vi "Client - Child 1 -  GET.vi"(8 "error in":errorcluster) -> (0 "error out":errorcluster, 2 "value":dbl)   [LabVIEW 2023, in "Client.lvlib" / "Client.lvclass"]
uses:
  Client.lvclass
  Child_1/Usr Ev/Child_1 - Ctrl - Enum - Events.ctl
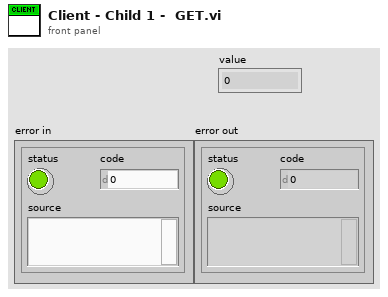
[diagram p1: front panel]
types:
  T1 = typedef "Actor_Child_1.lvlib/Child_1_Class.lvclass/Child_1 - Ctrl - Enum - Events.ctl" = enum16{"SEND MESSAGE Ev", "STOP_ACTOR Ev", "INIT_ACTOR Ev", "START Ev", "STOP Ev", "GET Ev", "SET Ev", "ERROR_HANDLER Ev", "RESET Ev", "T2 Ev", "T3 Ev", "T4 Ev"}
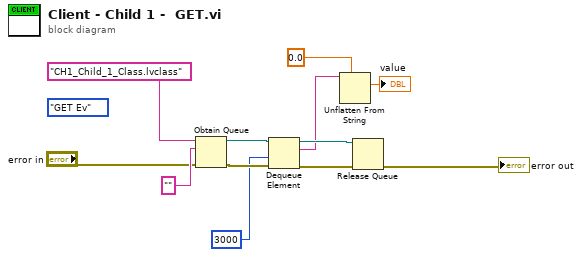
[diagram p0: block diagram]
diagram:
  (unwired) Child_1_-_Ctrl_-_Enum_-_Events."GET Ev" ("Events")
  n1 = Obtain Queue(name (unnamed)="CH1_Child_1_Class.lvclass", element data type="", error in (no error)="error in") -> (queue out=w9:refnum<queue>, error out=w10:errorcluster)  [unwired: 2 in, 1 out]
  n2 = Dequeue Element(queue=w9, timeout in ms (-1)=3000, error in (no error)=w10) -> (queue out=w6:refnum<queue>, element=w5:string, error out=w7:errorcluster)  [unwired: 1 out]
  n3 = Unflatten From String(type=0.0, binary string=w5) -> (value=→"value":dbl)  [unwired: 3 in, 2 out]
  n4 = Release Queue(queue=w6, error in (no error)=w7) -> (error out=→"error out":errorcluster)  [unwired: 1 in, 2 out]
